vi "IFile Write.vi"(8 "error in (no error)":errorcluster, 11 "INIScoreFile in":refnum<class "INIScoreFile.lvclass">) -> (0 "error out":errorcluster, 3 "INIScoreFile out":refnum<class "INIScoreFile.lvclass">)   [LabVIEW 2020, in "INIScoreFile.lvclass"]
uses:
  INIScoreFile.lvclass
  INIScoreFile.lvclass/INIScoreFile.ctl
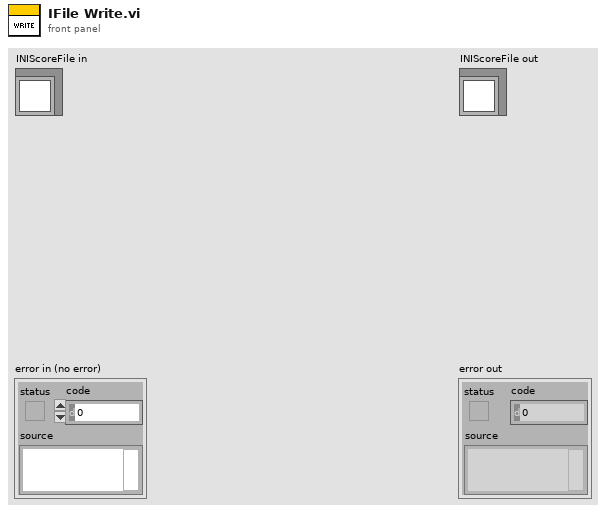
[diagram p1: front panel]
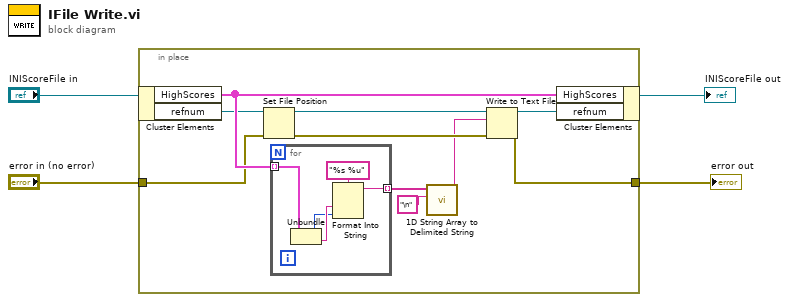
[diagram p0: block diagram]
diagram:
  n1 = in-place {
    in-place-border: "error in (no error)" -> [w10]
    in-place-border: [w5] -> w1
    n2 = in-place-cluster #1("INIScoreFile in") -> ("HighScores"=w14:cluster{"Score":u32, "Name":string}[], "refnum"=w11:refnum<file>)
    n3 = Set File Position(refnum=w11, error in=w10) -> (refnum out=w9:refnum<file>, error out=w8:errorcluster)  [unwired: 2 in]
    n4 = for {
      tunnel: w14 -> [w19] mode=indexing
      tunnel: [w17] -> w13 mode=indexing
      n5 = Unbundle(w19) -> ("Score"=w15:u32, "Name"=w16:string)
      n6 = Format Into String(format string="%s %u", w16, w15) -> (resulting string=w17:string)  [unwired: 2 in, 1 out]
    }
    n7 = call <vilib>:"1D String Array to Delimited String.vi"("delimiter"="\n", "string array"=w13) -> ("delimited string"=w7:string)  [unwired: 9 in]
    n8 = Write to Text File(file (use dialog)=w9, text=w7, error in=w8) -> (refnum out=w6:refnum<file>, error out=w5:errorcluster)  [unwired: 1 in, 1 out]
    n9 = in-place-cluster #1("HighScores"=w14, "refnum"=w6) -> (→"INIScoreFile out":refnum<class "INIScoreFile.lvclass">)
  }
  "error out" <- w1
